vi "Destroy.vi"(0 "reference":refnum<class "Grid.lvclass">, 5 "error in (no error)":errorcluster) -> (15 "# of objects":i32, 19 "error out":errorcluster)   [LabVIEW 2016, in "Grid.lvclass"]
doc: "Destroys an object created with a Grid constructor VI or a subclass of the Grid class. This VI must be reentrant.\n\n[GOOP 2.1]"
uses:
  <resource>/Framework/Providers/Open_GDS/UML/Grid_class/Grid.lvclass
panel:
  out "reference out":refnum<class "Grid.lvclass">
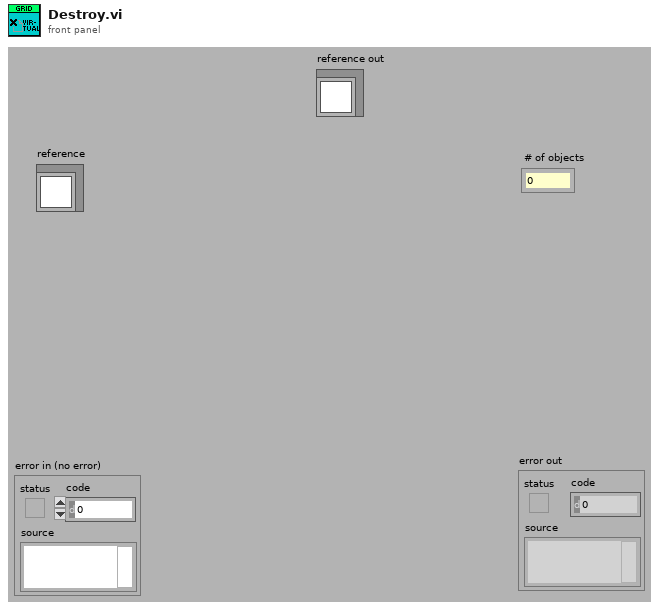
[diagram p1: front panel]
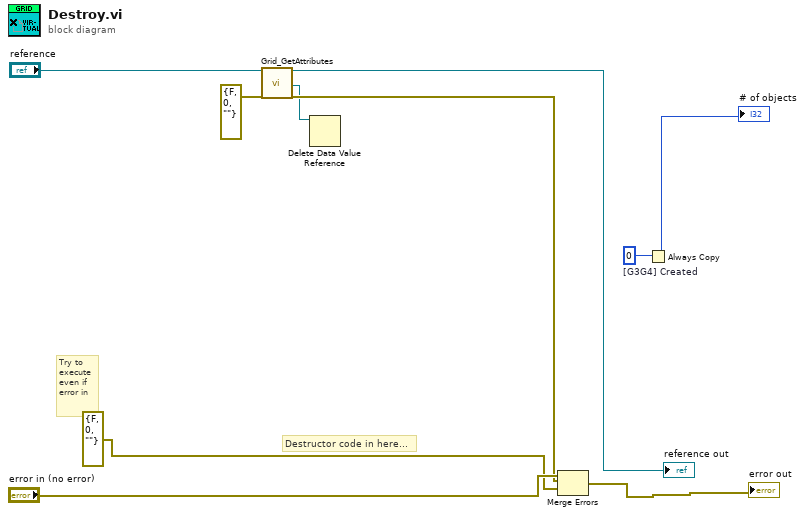
[diagram p0: block diagram]
diagram:
  w1 = 0  # [G3G4] Created
  # "Destructor code in here..."
  # "Try to\nexecute\neven if\nerror in"
  n1 = call <resource>:"Grid_GetAttributes.vi"("reference in"="reference", "error in (no error)"=errorcluster {"status"=FALSE, "code"=0, "source"=""}) -> ("reference out"=→"reference out":refnum<class "Grid.lvclass">, "DataRef"=w3:refnum<data-value>, "error out"=w5:errorcluster)  [unwired: 1 in, 14 out]
  n2 = Delete Data Value Reference(data value reference=w3) -> ()  [unwired: 1 in, 2 out]
  n3 = Merge Errors("error in (no error)", w5, errorcluster {"status"=FALSE, "code"=0, "source"=""} ("error in (no error)")) -> (→"error out":errorcluster)
  n4 = Always Copy(1:w1) -> (0:→"# of objects":i32)
